vi "SerialCommunicationTransport.vi"(6 "Configuration File Path":path, 7 "Queue Name In":string="firmata-serial-communication", 8 "error in":errorcluster, 9 "Baud Rate":u32(ring)=57600 items=["75"=75, "110"=110, "134"=134, "150"=150, "300"=300, "600"=600, "1200"=1200, "1800"=1800, "2400"=2400, "4800"=4800, "7200"=7200, "9600"=9600, "14400"=14400, "19200"=19200, "28800"=28800, "38400"=38400, "56000"=56000, "57600"=57600, "115200"=115200, "128000"=128000, "230400"=230400], 10 "Comport":refnum<visa-resource-name>="COM20", 11 "Firmata Message Event":refnum<user-event>) -> (0 "error out":errorcluster)   [LabVIEW 2020]
doc: "Serial Communication Engine. This VI will continuously run and service a queue from where it receives commands such as initialize, or cleanup and obviously \"send - receive\".\nBy default if nothing is received on the queue, the engine will monitor the transport medium for unsollicited messages and submit those over the notifier and user event bus (if one is provided)"
uses:
  Controls/Transport Notifier Response.ctl
  Controls/Transport Queue Message.ctl
  Controls/Transport Commands.ctl
  Controls/Transport Engine Loop Data.ctl
  Controls/SerialCommunicationConfigData.ctl
  <vilib>/Instr/_visa.llb/VISA Configure Serial Port (Instr).vi
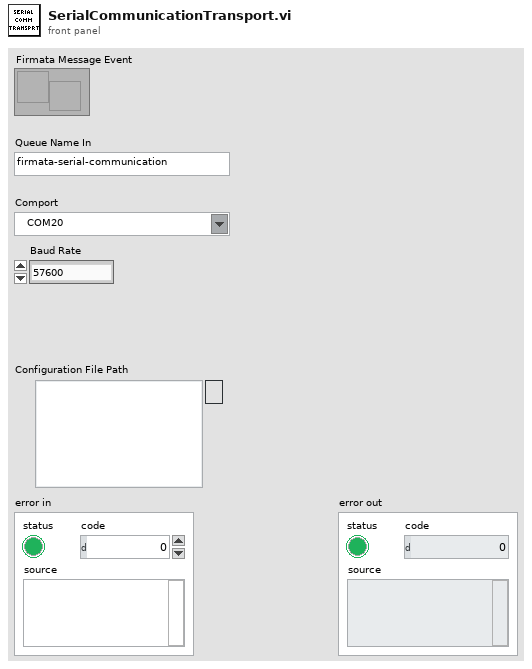
[diagram p1: front panel]
types:
  T1 = typedef "Transport Queue Message.ctl" = cluster{"Command":T2, "Message":u8[]}
  T2 = typedef "Transport Commands.ctl" = enum16{"Initialize", "Transmit - Receive", "Cleanup", "Cleanup And Stop"}
  T3 = typedef "Transport Engine Loop Data.ctl" = cluster{"Comport":refnum<visa-resource-name>, "Baud Rate":u32, "Configuration File Path":path, "Configuration Data":T4}
  T4 = typedef "SerialCommunicationConfigData.ctl" = cluster{"No Response Timeout Ms":u32, "Response Complete Timeout Ms":u32, "Max Rx Length":u32}
  T5 = typedef "Transport Notifier Response.ctl" = cluster{"Message":u8[], "Error":errorcluster}
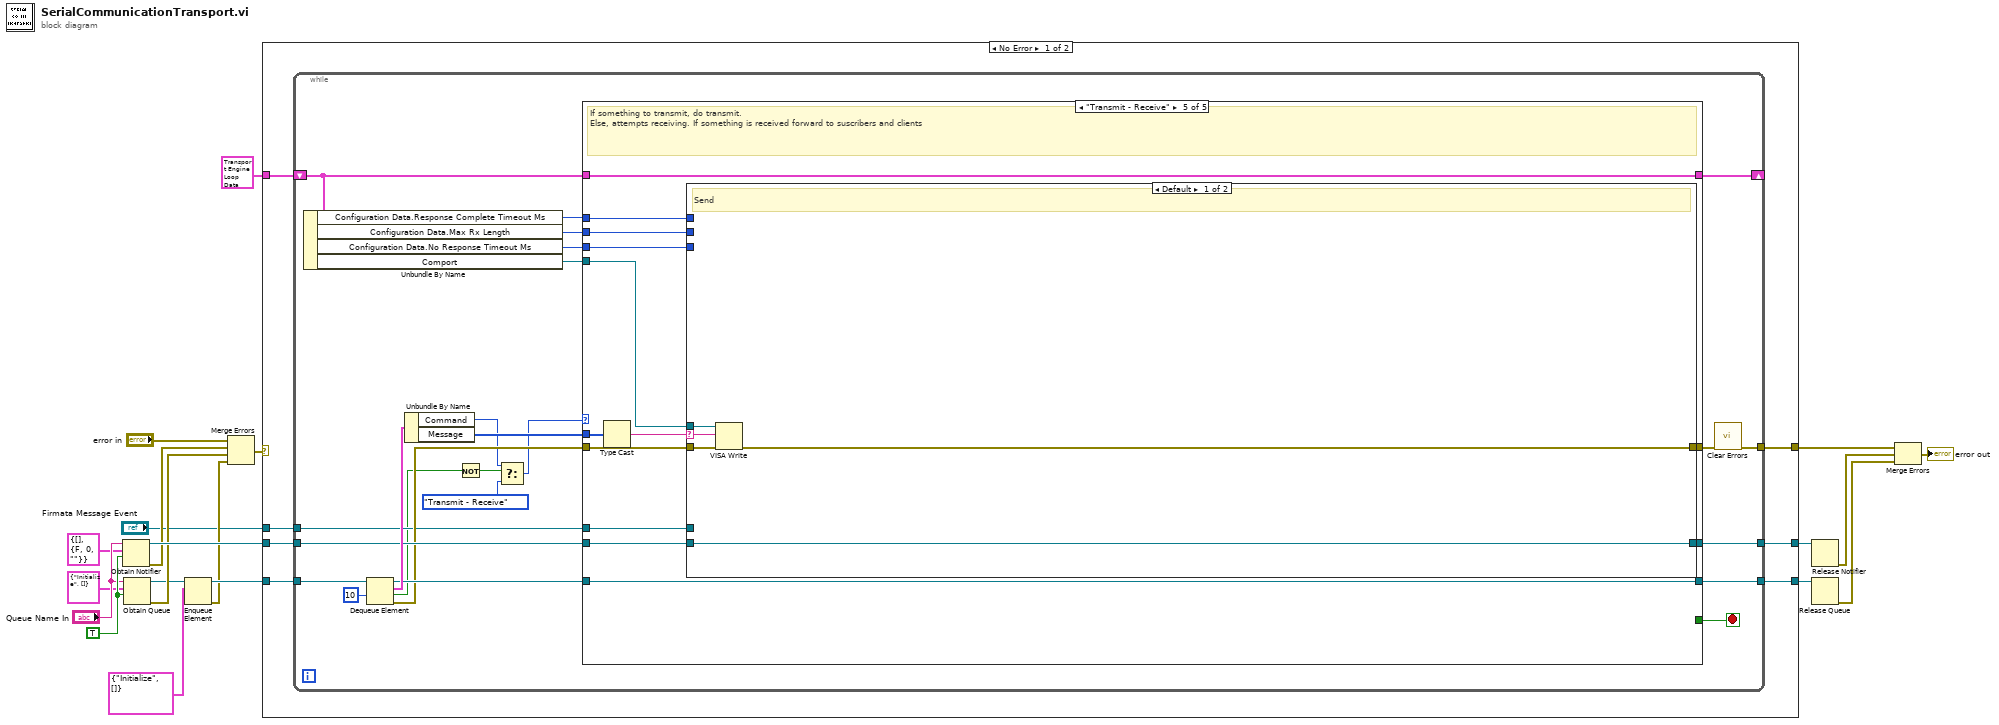
[diagram p0: block diagram]
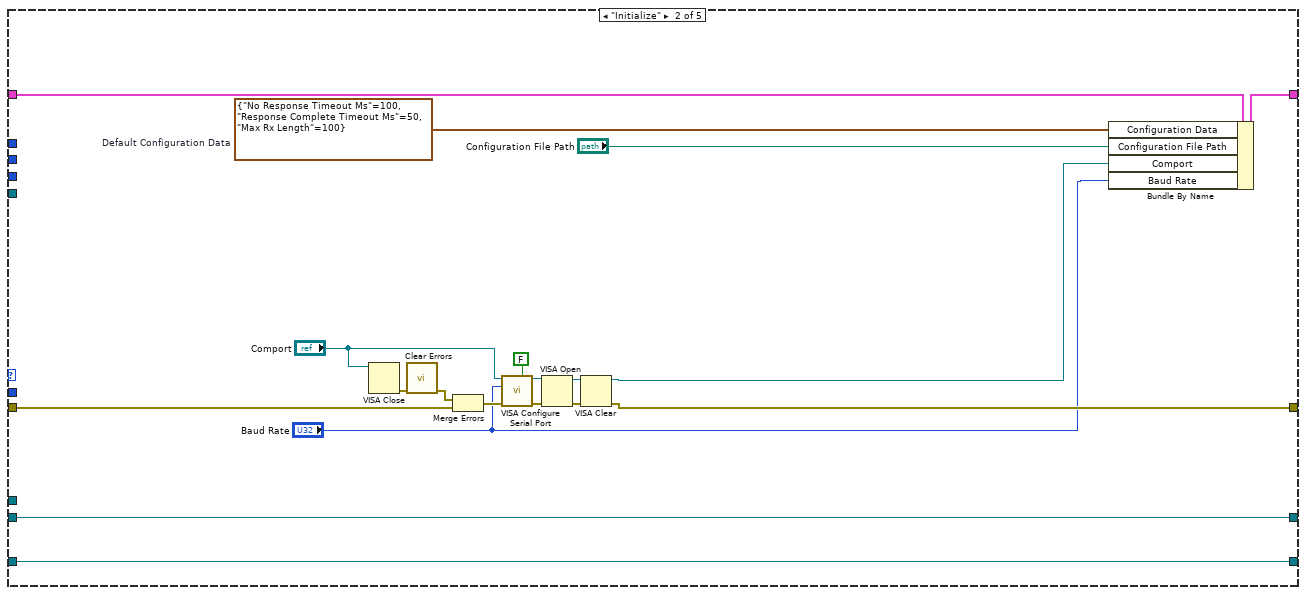
[diagram p3: hidden frame]
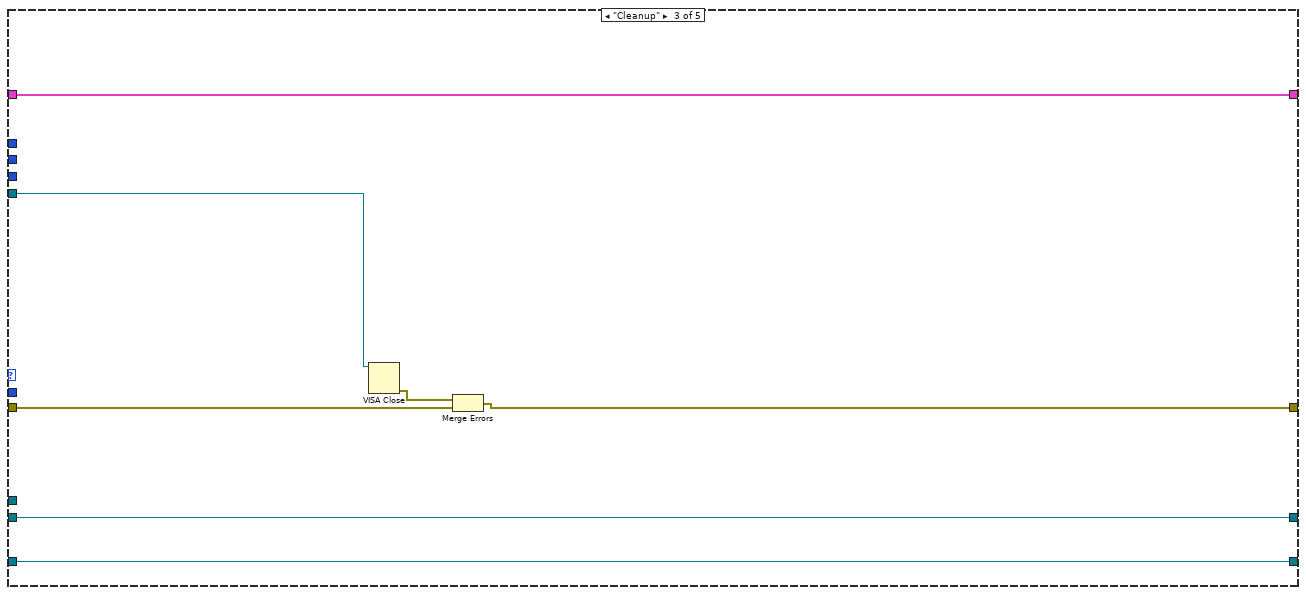
[diagram p4: hidden frame]
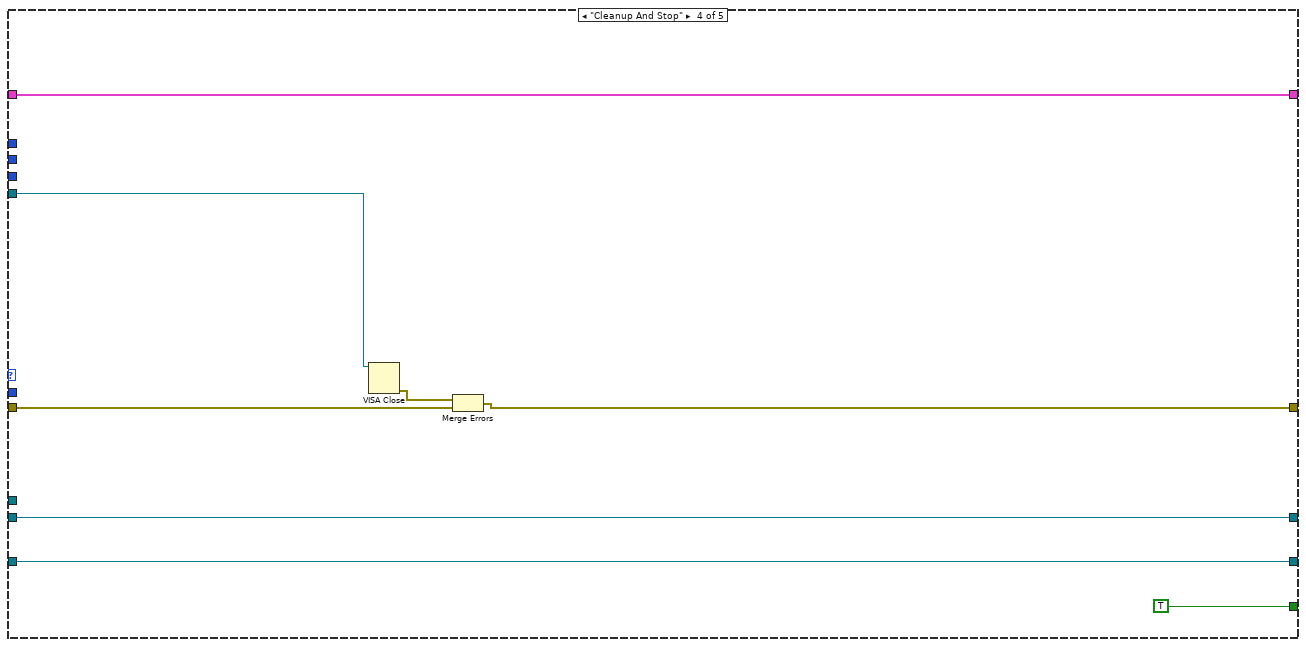
[diagram p5: hidden frame]
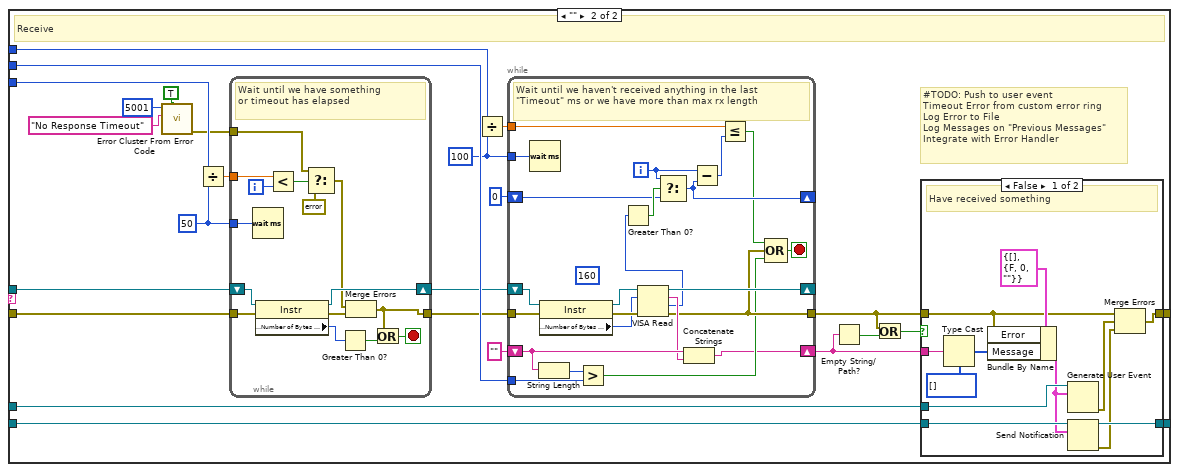
[diagram p6: hidden frame]
diagram:
  w21 = TRUE ("create if not found? (T)")
  n1 = Obtain Notifier(name (unnamed)="Queue Name In", notification data type=T5 {"Message"=[], "Error"={"status"=FALSE, "code"=0, "source"=""}} ("Transport Notifier Response"), create if not found? (T)=w21) -> (notifier out=w19:refnum<notifier>, error out=w8:errorcluster)  [unwired: 1 in, 1 out]
  n2 = Obtain Queue(name (unnamed)="Queue Name In", element data type=T1 {"Command"=enum."Initialize", "Message"=[]}, create if not found? (T)=w21) -> (queue out=w6:refnum<queue>, error out=w18:errorcluster)  [unwired: 2 in, 1 out]
  n3 = Enqueue Element(queue=w6, element=T1 {"Command"=enum."Initialize", "Message"=[]}) -> (queue out=w5:refnum<queue>, error out=w3:errorcluster)  [unwired: 2 in, 1 out]
  n4 = Merge Errors("error in", w8, w18, w3) -> (w17:errorcluster)
  n5 = case shown="No Error" w17 {
    selector: w17 -> [_ w185]
    tunnel: [w28 w185] -> w12
    tunnel: w5 -> [w27 w187]
    tunnel: w19 -> [w26 w186]
    tunnel: T3 {"Comport"="COM20", "Baud Rate"=57600, "Configuration File Path"=path "", "Configuration Data"={"No Response Timeout Ms"=5000, "Response Complete Timeout Ms"=200, "Max Rx Length"=1048}} ("Transport Engine Data") -> [w25 _]
    tunnel: [w24 w187] -> w14
    tunnel: [w23 w186] -> w13
    tunnel: "Firmata Message Event" -> [w22 _]
    frame No Error {
      n6 = while {
        tunnel: w27 -> [w52]
        tunnel: w26 -> [w43]
        shift-right: [w46] -> _
        shift-left: w25 -> [w41]
        tunnel: [w44] -> w24
        tunnel: [w42] -> w23
        tunnel: [w50] -> w28
        tunnel: w22 -> [w31]
        stop <- w47 stop-if-true
        n7 = Unbundle By Name(w41) -> ("Configuration Data.Response Complete Timeout Ms"=w37:u32, "Configuration Data.Max Rx Length"=w38:u32, "Configuration Data.No Response Timeout Ms"=w39:u32, "Comport"=w40:refnum<visa-resource-name>)
        n8 = Dequeue Element(queue=w52, timeout in ms (-1)=10) -> (queue out=w45:refnum<queue>, element=w49:T1, timed out?=w29:bool, error out=w36:errorcluster)  [unwired: 1 in]
        n9 = Unbundle By Name(w49) -> ("Command"=w34:T2, "Message"=w48:u8[])
        n10 = Not(x=w29) -> (.not. x?=w30:bool)
        n11 = Select(t=w34, s=w30, f=Transport_Commands."Transmit - Receive") -> (s? t:f=w33:T2)
        n12 = case shown="\"Transmit - Receive\"" w33 {
          tunnel: [w56 w63 w81 w89 w93] -> w51
          tunnel: w36 -> [w56 w66 w82 w90 w102]
          tunnel: w48 -> [_ _ _ _ w100]
          tunnel: [_ _ _ TRUE _] -> w47
          tunnel: w41 -> [w55 w60 w79 w87 w103]
          tunnel: [w55 w74 w79 w87 w103] -> w46
          tunnel: w45 -> [w54 w62 w78 w86 w96]
          tunnel: [w54 w62 w78 w86 w96] -> w44
          tunnel: w43 -> [w53 w61 w77 w85 w95]
          tunnel: [w53 w61 w77 w85 w94] -> w42
          tunnel: w40 -> [_ _ w76 w84 w101]
          tunnel: w39 -> [_ _ _ _ w99]
          tunnel: w38 -> [_ _ _ _ w98]
          tunnel: w37 -> [_ _ _ _ w97]
          tunnel: w31 -> [_ _ _ _ w92]
          frame Default {
          }
          frame "Initialize" {
            w57 = T4 {"No Response Timeout Ms"=100, "Response Complete Timeout Ms"=50, "Max Rx Length"=100}  # Default Configuration Data
            n13 = VISA Close(VISA resource name="Comport") -> (error out=w68:errorcluster)  [unwired: 1 in]
            n14 = call <vilib>:"Clear Errors.vi"("error in (no error)"=w68) -> ("error out"=w67:errorcluster)  [unwired: 5 in, 1 out]
            n15 = Merge Errors(w67, w66) -> (w65:errorcluster)
            n16 = call-poly "VISA Configure Serial Port"("VISA resource name"="Comport", "Enable Termination\nChar (T)"=FALSE ("Enable Termination\nChar (T)"), "baud rate (9600)"="Baud Rate", "error in (no error)"=w65) -> ("VISA resource name out"=w72:refnum<visa-resource-name>, "error out"=w73:errorcluster)  [unwired: 10 in]
            n17 = VISA Open(error in (no error)=w73, VISA resource name=w72) -> (VISA resource name=w70:refnum<visa-resource-name>, error out=w71:errorcluster)  [unwired: 3 in]
            n18 = VISA Clear(VISA resource name=w70, error in (no error)=w71) -> (VISA resource name out=w58:refnum<visa-resource-name>, error out=w63:errorcluster)
            n19 = Bundle By Name(cluster=w60, "Configuration Data"=w57, "Configuration File Path"="Configuration File Path", "Comport"=w58, "Baud Rate"="Baud Rate") -> (w74:T3)
          }
          frame "Cleanup" {
            n20 = VISA Close(VISA resource name=w76) -> (error out=w80:errorcluster)  [unwired: 1 in]
            n21 = Merge Errors(w80, w82) -> (w81:errorcluster)
          }
          frame "Cleanup And Stop" {
            n22 = VISA Close(VISA resource name=w84) -> (error out=w88:errorcluster)  [unwired: 1 in]
            n23 = Merge Errors(w88, w90) -> (w89:errorcluster)
          }
          frame "Transmit - Receive" {
            # "If something to transmit, do transmit.\nElse, attempts receiving. If something is received forward to suscribers and clients"
            n24 = Type Cast(x=w100) -> (*(type *) &x=w91:string)  [unwired: 1 in]
            n25 = case shown="Default" w91 {
              selector: w91 -> [w104 _]
              tunnel: w102 -> [w106 w132]
              tunnel: w101 -> [w105 w131]
              tunnel: w99 -> [_ w130]
              tunnel: w98 -> [_ w125]
              tunnel: w97 -> [_ w124]
              tunnel: w95 -> [w107 w115]
              tunnel: [w107 w114] -> w94
              tunnel: [w106 w113] -> w93
              tunnel: w92 -> [_ w112]
              frame Default {
                # "Send"
                n26 = VISA Write(VISA resource name=w105, write buffer=w104, error in (no error)=w106) -> ()  [unwired: 3 out]
              }
              frame "" {
                w120 = u32 100 ("milliseconds to wait")
                w122 = u32 50 ("milliseconds to wait")
                # "#TODO: Push to user event\nTimeout Error from custom error ring\nLog Error to File\nLog Messages on \"Previous Messages\"\nIntegrate with Error Handler"
                # "Receive"
                n27 = call <vilib>:"Error Cluster From Error Code.vi"("show call chain? (False)"=TRUE, "error message (\"\")"="No Response Timeout" ("error message (\"\")"), "error code (0)"=5001) -> ("error out"=w126:errorcluster)  [unwired: 6 in]
                n28 = Divide(x=w130, y=w122) -> (x/y=w121:dbl)
                n29 = while {
                  shift-right: [w183] -> w123
                  shift-left: w131 -> [w184]
                  tunnel: w122 -> [w181]
                  tunnel: w121 -> [w180]
                  tunnel: w132 -> [w177]
                  tunnel: [w170] -> w117
                  tunnel: w126 -> [w174]
                  i -> [w179]
                  stop <- w178 stop-if-true
                  # "Wait until we have something\nor timeout has elapsed"
                  n30 = Wait (ms)(milliseconds to wait=w181) -> ()  [unwired: 1 out]
                  n31 = property class="Instr"(reference=w184, error in=w177) -> (reference out=w183:refnum<visa-resource-name>, error out=w171:errorcluster, "Serial Settings:Number of Bytes at Serial Port"=w182:u32)
                  n32 = Less?(x=w180, y=w179) -> (x < y?=w175:bool)
                  n33 = Select(t=w174, s=w175, f=errorcluster {"status"=FALSE, "code"=0, "source"=""}) -> (s? t:f=w172:errorcluster)
                  n34 = Greater Than 0?(x=w182) -> (x > 0?=w176:bool)
                  n35 = Merge Errors(w172, w171) -> (w170:errorcluster)
                  n36 = Or(x=w170, y=w176) -> (x .or. y?=w178:bool)
                }
                n37 = Divide(x=w124, y=w120) -> (x/y=w119:dbl)
                n38 = while {
                  shift-right: [w169] -> _
                  shift-left: w123 -> [w166]
                  tunnel: w120 -> [w165]
                  tunnel: w119 -> [w160]
                  shift-right: [w161] -> _
                  shift-left: 0 -> [w163]
                  tunnel: w117 -> [w158]
                  tunnel: [w152] -> w111
                  tunnel: w125 -> [w156]
                  shift-right: [w149] -> w109
                  shift-left: "" -> [w155]
                  i -> [w162]
                  stop <- w150 stop-if-true
                  (unwired) u32 160 ("byte count")
                  # "Wait until we haven't received anything in the last \"Timeout\" ms or we have more than max rx length"
                  n39 = Wait (ms)(milliseconds to wait=w165) -> ()  [unwired: 1 out]
                  n40 = String Length(string=w155) -> (length=w157:i32)
                  n41 = property class="Instr"(reference=w166, error in=w158) -> (reference out=w167:refnum<visa-resource-name>, error out=w168:errorcluster, "Serial Settings:Number of Bytes at Serial Port"=w147:u32)
                  n42 = Greater?(x=w157, y=w156) -> (0:w151:bool)
                  n43 = VISA Read(VISA resource name=w167, byte count=w147, error in (no error)=w168) -> (VISA resource name out=w169:refnum<visa-resource-name>, read buffer=w154:string, return count=w148:u32, error out=w152:errorcluster)
                  n44 = Greater Than 0?(x=w148) -> (x > 0?=w164:bool)
                  n45 = Select(t=w162, s=w164, f=w163) -> (s? t:f=w161:i32)
                  n46 = Concatenate Strings(w155, w154) -> (w149:string)
                  n47 = Subtract(x=w162, y=w161) -> (x-y=w159:i32)
                  n48 = Less Or Equal?(x=w160, y=w159) -> (x <= y?=w153:bool)
                  n49 = Compound Arithmetic op=OR(w153, w152, w151) -> (w150:bool)
                }
                n50 = Empty String/Path?(string/path=w109) -> (empty?=w110:bool)
                n51 = Or(x=w111, y=w110) -> (x .or. y?=w108:bool)
                n52 = case shown="False" w108 {
                  tunnel: w109 -> [w143 _]
                  tunnel: w115 -> [w142 w145]
                  tunnel: [w141 w145] -> w114
                  tunnel: w111 -> [w138 w146]
                  tunnel: [w137 w146] -> w113
                  tunnel: w112 -> [w136 _]
                  frame False {
                    # "Have received something"
                    n53 = Type Cast(type=u8[] [] ("Message"), x=w143) -> (*(type *) &x=w140:u8[])
                    n54 = Bundle By Name(cluster=T5 {"Message"=[], "Error"={"status"=FALSE, "code"=0, "source"=""}} ("notification"), "Error"=w138, "Message"=w140) -> (w135:T5)
                    n55 = Generate User Event(user event=w136, event data cluster=w135) -> (error out=w133:errorcluster)  [unwired: 2 in, 1 out]
                    n56 = Send Notification(notification=w135, notifier=w142) -> (notifier out=w141:refnum<notifier>, error out=w134:errorcluster)  [unwired: 1 in]
                    n57 = Merge Errors(w138, w133, w134) -> (w137:errorcluster)
                  }
                  frame True {
                    # "Nothing Received"
                  }
                }
              }
            }
          }
        }
        n58 = call <vilib>:"Clear Errors.vi"("error in (no error)"=w51) -> ("error out"=w50:errorcluster)  [unwired: 5 in, 1 out]
      }
    }
    frame Error {
    }
  }
  n59 = Release Notifier(notifier=w13) -> (error out=w10:errorcluster)  [unwired: 2 in, 2 out]
  n60 = Release Queue(queue=w14) -> (error out=w9:errorcluster)  [unwired: 2 in, 2 out]
  n61 = Merge Errors(w12, w10, w9) -> (→"error out":errorcluster)
